vi "S4GUI.vi"(7 "Tab ObsEng":enum32{"Obs", "CCD modes", "Guider", "Eng"}(tab)) -> ()   [LabVIEW 2018] (continued)
        n3771 = call-dynamic "Write # Images.vi"("error in (no error)"=w8549, "# Images"="Exp ch3", "Interface in"=w8552) -> ("error out"=w8497:errorcluster, "Interface out"=w8500:refnum<class "Interface.lvclass">)  [unwired: 7 in]
        n3772 = call-dynamic "ValidateExp.vi"("error in (no error)"=w8497, "Interface in"=w8500) -> ("error out"=w8496:errorcluster, "Interface out"=w8499:refnum<class "Interface.lvclass">)  [unwired: 8 in]
        n3773 = call-dynamic "Read # Images.vi"("error in (no error)"=w8496, "Interface in"=w8499) -> ("error out"=w8495:errorcluster, "# Images"=w8494:u32, "Interface out"=w8498:refnum<class "Interface.lvclass">)  [unwired: 7 in]
        n3774 = call-dynamic "Write #PREV Images.vi"("error in (no error)"=w8495, "#PREV FRAMES"=w8494, "Interface in"=w8498) -> ("error out"=w8548:errorcluster, "Interface out"=w8547:refnum<class "Interface.lvclass">)  [unwired: 7 in]
        n3775 = call-dynamic "Write Interface.vi"("error in (no error)"=w8548, "Interface.lvclass"=w8547, "Channel in"=w8554) -> ("error out"=w8546:errorcluster, "Channel out"=w8553:refnum<class "Channel.lvclass">)  [unwired: 7 in]
        n3776 = property on="Exposures Done ch3" class="Slide (strict)"("Scale.Maximum"=w8494, "Scale.Minimum"=0.0 ("Scale.Range:Minimum")) -> ()  [unwired: 2 in, 2 out]
        n3777 = local write "Exp ch3"(w8494) -> ()
        n3778 = call-dynamic "Write Channel.vi"("error in (no error)"=w8546, "Channel.lvclass"=w8553, "Acquisition in"=w8556) -> ("error out"=w8545:errorcluster, "Acquisition out"=w8555:refnum<class "Acquisition.lvclass">)  [unwired: 7 in]
        n3779 = call-dynamic "Write AcquisitionC.vi"("error in (no error)"=w8545, "Acquisition.lvclass"=w8555, "S4ACS_GUI in"=w8559) -> ("error out"=w8528:errorcluster, "S4ACS_GUI out"=w8529:refnum<class "S4GUI.lvclass">)  [unwired: 7 in]
        n3780 = call-dynamic "Read AcquisitionD.vi"("error in (no error)"=w8528, "S4ACS_GUI in"=w8529) -> ("error out"=w8535:errorcluster, "Acquisition.lvclass"=w8543:refnum<class "Acquisition.lvclass">, "S4ACS_GUI out"=w8544:refnum<class "S4GUI.lvclass">)  [unwired: 7 in]
        n3781 = call-dynamic "Read Channel.vi"("error in (no error)"=w8535, "Acquisition in"=w8543) -> ("error out"=w8536:errorcluster, "Channel.lvclass"=w8542:refnum<class "Channel.lvclass">, "Acquisition out"=w8541:refnum<class "Acquisition.lvclass">)  [unwired: 7 in]
        n3782 = call-dynamic "Read Interface.vi"("error in (no error)"=w8536, "Channel in"=w8542) -> ("error out"=w8534:errorcluster, "Interface.lvclass"=w8537:refnum<class "Interface.lvclass">, "Channel out"=w8539:refnum<class "Channel.lvclass">)  [unwired: 7 in]
        n3783 = call-dynamic "Write # Images.vi"("error in (no error)"=w8534, "# Images"="Exp ch4", "Interface in"=w8537) -> ("error out"=w8488:errorcluster, "Interface out"=w8490:refnum<class "Interface.lvclass">)  [unwired: 7 in]
        n3784 = call-dynamic "ValidateExp.vi"("error in (no error)"=w8488, "Interface in"=w8490) -> ("error out"=w8487:errorcluster, "Interface out"=w8489:refnum<class "Interface.lvclass">)  [unwired: 8 in]
        n3785 = call-dynamic "Read # Images.vi"("error in (no error)"=w8487, "Interface in"=w8489) -> ("error out"=w8492:errorcluster, "# Images"=w8491:u32, "Interface out"=w8493:refnum<class "Interface.lvclass">)  [unwired: 7 in]
        n3786 = call-dynamic "Write #PREV Images.vi"("error in (no error)"=w8492, "#PREV FRAMES"=w8491, "Interface in"=w8493) -> ("error out"=w8533:errorcluster, "Interface out"=w8532:refnum<class "Interface.lvclass">)  [unwired: 7 in]
        n3787 = property on="Exposures Done ch4" class="Slide (strict)"("Scale.Maximum"=w8491, "Scale.Minimum"=0.0 ("Scale.Range:Minimum")) -> ()  [unwired: 2 in, 2 out]
        n3788 = local write "Exp ch4"(w8491) -> ()
        n3789 = call-dynamic "Write Interface.vi"("error in (no error)"=w8533, "Interface.lvclass"=w8532, "Channel in"=w8539) -> ("error out"=w8531:errorcluster, "Channel out"=w8538:refnum<class "Channel.lvclass">)  [unwired: 7 in]
        n3790 = call-dynamic "Write Channel.vi"("error in (no error)"=w8531, "Channel.lvclass"=w8538, "Acquisition in"=w8541) -> ("error out"=w8530:errorcluster, "Acquisition out"=w8540:refnum<class "Acquisition.lvclass">)  [unwired: 7 in]
        n3791 = call-dynamic "Write AcquisitionD.vi"("error in (no error)"=w8530, "Acquisition.lvclass"=w8540, "S4ACS_GUI in"=w8544) -> ("error out"=w8522:errorcluster, "S4ACS_GUI out"=w8523:refnum<class "S4GUI.lvclass">)  [unwired: 7 in]
      }
      event "#cycles ch1": Value Change {
        n3792 = event-data() -> ("NewVal"=w8593:u32)  [unwired: 1 in]
        n3793 = call-dynamic "Read AcquisitionA.vi"("error in (no error)"=w8615, "S4ACS_GUI in"=w8616) -> ("error out"=w8610:errorcluster, "Acquisition.lvclass"=w8613:refnum<class "Acquisition.lvclass">, "S4ACS_GUI out"=w8614:refnum<class "S4GUI.lvclass">)  [unwired: 7 in]
        n3794 = call-dynamic "Read Channel.vi"("error in (no error)"=w8610, "Acquisition in"=w8613) -> ("error out"=w8607:errorcluster, "Channel.lvclass"=w8606:refnum<class "Channel.lvclass">, "Acquisition out"=w8612:refnum<class "Acquisition.lvclass">)  [unwired: 7 in]
        n3795 = call-dynamic "Write ciclos.vi"("error in (no error)"=w8607, "ciclos"=w8593, "Channel in"=w8606) -> ("error out"=w8604:errorcluster, "Channel out"=w8605:refnum<class "Channel.lvclass">)  [unwired: 7 in]
        n3796 = call-dynamic "Write prev ciclos.vi"("error in (no error)"=w8604, "prev ciclos"=w8593, "Channel in"=w8605) -> ("error out"=w8602:errorcluster, "Channel out"=w8603:refnum<class "Channel.lvclass">)  [unwired: 7 in]
        n3797 = property on="Cycles Done ch1" class="Slide (strict)"("Scale.Maximum"=w8593, "Scale.Minimum"=0.0 ("Scale.Range:Minimum")) -> ()  [unwired: 2 in, 2 out]
        n3798 = call-dynamic "Write Channel.vi"("error in (no error)"=w8602, "Channel.lvclass"=w8603, "Acquisition in"=w8612) -> ("error out"=w8609:errorcluster, "Acquisition out"=w8611:refnum<class "Acquisition.lvclass">)  [unwired: 7 in]
        n3799 = call-dynamic "Write AcquisitionA.vi"("error in (no error)"=w8609, "Acquisition.lvclass"=w8611, "S4ACS_GUI in"=w8614) -> ("error out"=w8600:errorcluster, "S4ACS_GUI out"=w8601:refnum<class "S4GUI.lvclass">)  [unwired: 7 in]
        n3800 = call-dynamic "Write ciclos.vi"("error in (no error)"=w8600, "ciclos"=w8593, "S4ACS_GUI in"=w8601) -> ("error out"=w8595:errorcluster, "S4ACS_GUI out"=w8597:refnum<class "S4GUI.lvclass">)  [unwired: 7 in]
        n3801 = call-dynamic "Write prev sequencias.vi"("error in (no error)"=w8595, "prev sequencias"=w8593, "S4GUI in"=w8597) -> ("error out"=w8594:errorcluster, "S4GUI out"=w8596:refnum<class "S4GUI.lvclass">)  [unwired: 7 in]
        n3802 = call-dynamic "Write TotalCiclos.vi"("error in (no error)"=w8594, "TotalCiclos"=w8593, "S4GUI in"=w8596) -> ("error out"=w8598:errorcluster, "S4GUI out"=w8599:refnum<class "S4GUI.lvclass">)  [unwired: 7 in]
      }
      event "#cycles ch2": Value Change {
        n3803 = event-data() -> ("NewVal"=w8617:u32)  [unwired: 1 in]
        n3804 = call "Read AcquisitionB.vi"("error in (no error)"=w8639, "S4ACS_GUI in"=w8640) -> ("error out"=w8634:errorcluster, "Acquisition.lvclass"=w8637:refnum<class "Acquisition.lvclass">, "S4ACS_GUI out"=w8638:refnum<class "S4GUI.lvclass">)  [unwired: 7 in]
        n3805 = call-dynamic "Read Channel.vi"("error in (no error)"=w8634, "Acquisition in"=w8637) -> ("error out"=w8632:errorcluster, "Channel.lvclass"=w8631:refnum<class "Channel.lvclass">, "Acquisition out"=w8636:refnum<class "Acquisition.lvclass">)  [unwired: 7 in]
        n3806 = call-dynamic "Write ciclos.vi"("error in (no error)"=w8632, "ciclos"=w8617, "Channel in"=w8631) -> ("error out"=w8629:errorcluster, "Channel out"=w8630:refnum<class "Channel.lvclass">)  [unwired: 7 in]
        n3807 = call-dynamic "Write prev ciclos.vi"("error in (no error)"=w8629, "prev ciclos"=w8617, "Channel in"=w8630) -> ("error out"=w8627:errorcluster, "Channel out"=w8628:refnum<class "Channel.lvclass">)  [unwired: 7 in]
        n3808 = call-dynamic "Write Channel.vi"("error in (no error)"=w8627, "Channel.lvclass"=w8628, "Acquisition in"=w8636) -> ("error out"=w8633:errorcluster, "Acquisition out"=w8635:refnum<class "Acquisition.lvclass">)  [unwired: 7 in]
        n3809 = property on="Cycles Done ch2" class="Slide (strict)"("Scale.Maximum"=w8617, "Scale.Minimum"=0.0 ("Scale.Range:Minimum")) -> ()  [unwired: 2 in, 2 out]
        n3810 = call "Write AcquisitionB.vi"("error in (no error)"=w8633, "Acquisition.lvclass"=w8635, "S4ACS_GUI in"=w8638) -> ("error out"=w8625:errorcluster, "S4ACS_GUI out"=w8626:refnum<class "S4GUI.lvclass">)  [unwired: 7 in]
        n3811 = call-dynamic "Write ciclos.vi"("error in (no error)"=w8625, "ciclos"=w8617, "S4ACS_GUI in"=w8626) -> ("error out"=w8620:errorcluster, "S4ACS_GUI out"=w8622:refnum<class "S4GUI.lvclass">)  [unwired: 7 in]
        n3812 = call-dynamic "Write prev sequencias.vi"("error in (no error)"=w8620, "prev sequencias"=w8617, "S4GUI in"=w8622) -> ("error out"=w8619:errorcluster, "S4GUI out"=w8621:refnum<class "S4GUI.lvclass">)  [unwired: 7 in]
        n3813 = call-dynamic "Write TotalCiclos.vi"("error in (no error)"=w8619, "TotalCiclos"=w8617, "S4GUI in"=w8621) -> ("error out"=w8623:errorcluster, "S4GUI out"=w8624:refnum<class "S4GUI.lvclass">)  [unwired: 7 in]
      }
      event "#cycles ch3": Value Change {
        n3814 = event-data() -> ("NewVal"=w8641:u32)  [unwired: 1 in]
        n3815 = call-dynamic "Read AcquisitionC.vi"("error in (no error)"=w8663, "S4ACS_GUI in"=w8664) -> ("error out"=w8658:errorcluster, "Acquisition.lvclass"=w8661:refnum<class "Acquisition.lvclass">, "S4ACS_GUI out"=w8662:refnum<class "S4GUI.lvclass">)  [unwired: 7 in]
        n3816 = call-dynamic "Read Channel.vi"("error in (no error)"=w8658, "Acquisition in"=w8661) -> ("error out"=w8656:errorcluster, "Channel.lvclass"=w8655:refnum<class "Channel.lvclass">, "Acquisition out"=w8660:refnum<class "Acquisition.lvclass">)  [unwired: 7 in]
        n3817 = call-dynamic "Write ciclos.vi"("error in (no error)"=w8656, "ciclos"=w8641, "Channel in"=w8655) -> ("error out"=w8653:errorcluster, "Channel out"=w8654:refnum<class "Channel.lvclass">)  [unwired: 7 in]
        n3818 = call-dynamic "Write prev ciclos.vi"("error in (no error)"=w8653, "prev ciclos"=w8641, "Channel in"=w8654) -> ("error out"=w8651:errorcluster, "Channel out"=w8652:refnum<class "Channel.lvclass">)  [unwired: 7 in]
        n3819 = call-dynamic "Write Channel.vi"("error in (no error)"=w8651, "Channel.lvclass"=w8652, "Acquisition in"=w8660) -> ("error out"=w8657:errorcluster, "Acquisition out"=w8659:refnum<class "Acquisition.lvclass">)  [unwired: 7 in]
        n3820 = property on="Cycles Done ch3" class="Slide (strict)"("Scale.Maximum"=w8641, "Scale.Minimum"=0.0 ("Scale.Range:Minimum")) -> ()  [unwired: 2 in, 2 out]
        n3821 = call-dynamic "Write AcquisitionC.vi"("error in (no error)"=w8657, "Acquisition.lvclass"=w8659, "S4ACS_GUI in"=w8662) -> ("error out"=w8649:errorcluster, "S4ACS_GUI out"=w8650:refnum<class "S4GUI.lvclass">)  [unwired: 7 in]
        n3822 = call-dynamic "Write ciclos.vi"("error in (no error)"=w8649, "ciclos"=w8641, "S4ACS_GUI in"=w8650) -> ("error out"=w8644:errorcluster, "S4ACS_GUI out"=w8646:refnum<class "S4GUI.lvclass">)  [unwired: 7 in]
        n3823 = call-dynamic "Write prev sequencias.vi"("error in (no error)"=w8644, "prev sequencias"=w8641, "S4GUI in"=w8646) -> ("error out"=w8643:errorcluster, "S4GUI out"=w8645:refnum<class "S4GUI.lvclass">)  [unwired: 7 in]
        n3824 = call-dynamic "Write TotalCiclos.vi"("error in (no error)"=w8643, "TotalCiclos"=w8641, "S4GUI in"=w8645) -> ("error out"=w8647:errorcluster, "S4GUI out"=w8648:refnum<class "S4GUI.lvclass">)  [unwired: 7 in]
      }
      event "#cycles ch4": Value Change {
        n3825 = event-data() -> ("NewVal"=w8665:u32)  [unwired: 1 in]
        n3826 = call-dynamic "Read AcquisitionD.vi"("error in (no error)"=w8687, "S4ACS_GUI in"=w8688) -> ("error out"=w8682:errorcluster, "Acquisition.lvclass"=w8685:refnum<class "Acquisition.lvclass">, "S4ACS_GUI out"=w8686:refnum<class "S4GUI.lvclass">)  [unwired: 7 in]
        n3827 = call-dynamic "Read Channel.vi"("error in (no error)"=w8682, "Acquisition in"=w8685) -> ("error out"=w8680:errorcluster, "Channel.lvclass"=w8679:refnum<class "Channel.lvclass">, "Acquisition out"=w8684:refnum<class "Acquisition.lvclass">)  [unwired: 7 in]
        n3828 = call-dynamic "Write ciclos.vi"("error in (no error)"=w8680, "ciclos"=w8665, "Channel in"=w8679) -> ("error out"=w8677:errorcluster, "Channel out"=w8678:refnum<class "Channel.lvclass">)  [unwired: 7 in]
        n3829 = call-dynamic "Write prev ciclos.vi"("error in (no error)"=w8677, "prev ciclos"=w8665, "Channel in"=w8678) -> ("error out"=w8675:errorcluster, "Channel out"=w8676:refnum<class "Channel.lvclass">)  [unwired: 7 in]
        n3830 = call-dynamic "Write Channel.vi"("error in (no error)"=w8675, "Channel.lvclass"=w8676, "Acquisition in"=w8684) -> ("error out"=w8681:errorcluster, "Acquisition out"=w8683:refnum<class "Acquisition.lvclass">)  [unwired: 7 in]
        n3831 = call-dynamic "Write AcquisitionD.vi"("error in (no error)"=w8681, "Acquisition.lvclass"=w8683, "S4ACS_GUI in"=w8686) -> ("error out"=w8673:errorcluster, "S4ACS_GUI out"=w8674:refnum<class "S4GUI.lvclass">)  [unwired: 7 in]
        n3832 = property on="Cycles Done ch4" class="Slide (strict)"("Scale.Maximum"=w8665, "Scale.Minimum"=0.0 ("Scale.Range:Minimum")) -> ()  [unwired: 2 in, 2 out]
        n3833 = call-dynamic "Write ciclos.vi"("error in (no error)"=w8673, "ciclos"=w8665, "S4ACS_GUI in"=w8674) -> ("error out"=w8668:errorcluster, "S4ACS_GUI out"=w8670:refnum<class "S4GUI.lvclass">)  [unwired: 7 in]
        n3834 = call-dynamic "Write prev sequencias.vi"("error in (no error)"=w8668, "prev sequencias"=w8665, "S4GUI in"=w8670) -> ("error out"=w8667:errorcluster, "S4GUI out"=w8669:refnum<class "S4GUI.lvclass">)  [unwired: 7 in]
        n3835 = call-dynamic "Write TotalCiclos.vi"("error in (no error)"=w8667, "TotalCiclos"=w8665, "S4GUI in"=w8669) -> ("error out"=w8671:errorcluster, "S4GUI out"=w8672:refnum<class "S4GUI.lvclass">)  [unwired: 7 in]
      }
      event "Start ch2": Value Change {
        n3836 = event-data() -> ()  [unwired: 1 in, 6 out]
        n3837 = call "Read Instrument.lvclass.vi"("error in (no error)"=w8702, "S4ACS_GUI in"=w8703) -> ("error out"=w8704:errorcluster, "Instrument.lvclass"=w8705:refnum<class "Instrument.lvclass">, "S4ACS_GUI out"=w8701:refnum<class "S4GUI.lvclass">)  [unwired: 7 in]
        n3838 = call-dynamic "Read mode.vi"("error in (no error)"=w8704, "Instrument in"=w8705) -> ("error out"=w8700:errorcluster, "mode"=w8699:bool)  [unwired: 7 in, 1 out]
        n3839 = call "Read AcquisitionB.vi"("error in (no error)"=w8700, "S4ACS_GUI in"=w8701) -> ("error out"=w8717:errorcluster, "Acquisition.lvclass"=w8718:refnum<class "Acquisition.lvclass">, "S4ACS_GUI out"=w8720:refnum<class "S4GUI.lvclass">)  [unwired: 7 in]
        n3840 = call-dynamic "Read Acq_state.vi"("error in (no error)"=w8717, "Acquisition in"=w8718) -> ("error out"=w8714:errorcluster, "Acq_state"=w8716:u32, "Acquisition out"=w8713:refnum<class "Acquisition.lvclass">)  [unwired: 7 in]
        n3841 = Not Equal?(x=w8716, y=u32 400) -> (x != y?=w8719:bool)
        n3842 = case shown="True" w8719 {
          tunnel: w8720 -> [w8733 w8772]
          tunnel: [w8733 w8764] -> w8712
          tunnel: [w8728 w8754] -> w8698
          tunnel: w8714 -> [w8735 w8762]
          tunnel: w8713 -> [w8738 w8765]
          tunnel: [w8729 w8753] -> w8711
          tunnel: w8710 -> [_ w8786]
          tunnel: w8709 -> [_ w8785]
          tunnel: w8708 -> [_ w8784]
          tunnel: w8707 -> [_ w8783]
          tunnel: w8706 -> [_ w8777]
          tunnel: w8699 -> [_ _]
          tunnel: w8697 -> [_ w8760]
          tunnel: w8696 -> [_ w8759]
          tunnel: w8695 -> [_ w8758]
          tunnel: w8694 -> [_ w8757]
          frame False {
            n3843 = call-dynamic "Read Acq_prevstate.vi"("error in (no error)"=w8735, "Acquisition in"=w8738) -> ("error out"=w8734:errorcluster, "Acq_prevstate"=w8736:u32, "Acquisition out"=w8737:refnum<class "Acquisition.lvclass">)  [unwired: 7 in]
            n3844 = call-dynamic "Write Acq_state.vi"("error in (no error)"=w8734, "Acq_state"=w8736, "Acquisition in"=w8737) -> ("error out"=w8725:errorcluster, "Acquisition out"=w8727:refnum<class "Acquisition.lvclass">)  [unwired: 7 in]
            n3845 = call-dynamic "Read enabled.vi"("error in (no error)"=w8725, "Server in"=w8727) -> ("error out"=w8724:errorcluster, "enabled"=w8721:bool, "Server out"=w8726:refnum<class "Acquisition.lvclass">)  [unwired: 7 in]
            n3846 = call-dynamic "Read Channel.vi"("error in (no error)"=w8724, "Acquisition in"=w8726) -> ("error out"=w8722:errorcluster, "Channel.lvclass"=w8723:refnum<class "Channel.lvclass">, "Acquisition out"=w8732:refnum<class "Acquisition.lvclass">)  [unwired: 7 in]
            n3847 = case shown="True" w8721 {
              tunnel: w8723 -> [w8740 w8750]
              tunnel: [w8740 w8748] -> w8731
              tunnel: w8722 -> [w8739 w8745]
              tunnel: [w8739 w8743] -> w8730
              frame False {
              }
              frame True {
                n3848 = call-dynamic "Read State Machine.vi"("error in (no error)"=w8745, "Device in"=w8750) -> ("error out"=w8741:errorcluster, "State Machine.lvclass"=w8742:refnum<class "State Machine.lvclass">, "Device out"=w8749:refnum<class "Channel.lvclass">)  [unwired: 7 in]
                n3849 = call "Next State.vi"("error in (no error)"=w8741, "New_State"=96, "State Machine in"=w8742) -> ("error out"=w8744:errorcluster, "State Machine out"=w8747:refnum<class "State Machine.lvclass">)  [unwired: 7 in]
                n3850 = call-dynamic "Write State Machine.vi"("error in (no error)"=w8744, "State Machine.lvclass"=w8747, "Device in"=w8749) -> ("error out"=w8743:errorcluster, "Device out"=w8748:refnum<class "Channel.lvclass">)  [unwired: 7 in]
              }
            }
            n3851 = call-dynamic "Write Channel.vi"("error in (no error)"=w8730, "Channel.lvclass"=w8731, "Acquisition in"=w8732) -> ("error out"=w8728:errorcluster, "Acquisition out"=w8729:refnum<class "Acquisition.lvclass">)  [unwired: 7 in]
          }
          frame True {
            # "obs type"
            # "suffix"
            # "object"
            n3852 = call "Read Instrument.lvclass.vi"("S4ACS_GUI in"=w8772) -> ("error out"=w8774:errorcluster, "Instrument.lvclass"=w8776:refnum<class "Instrument.lvclass">, "S4ACS_GUI out"=w8766:refnum<class "S4GUI.lvclass">)  [unwired: 8 in]
            n3853 = call "Read WPROT.vi"("error in (no error)"=w8774, "Instrument in"=w8776) -> ("error out"=w8773:errorcluster, "Opt_Selector.lvclass"=w8775:refnum<class "Opt_Selector.lvclass">)  [unwired: 7 in, 1 out]
            n3854 = call-dynamic "Read sequencia.vi"("error in (no error)"=w8773, "Opt_Selector in"=w8775) -> ()  [unwired: 7 in, 3 out]
            n3855 = case shown="Default" w8760 {
              tunnel: [u32 271 ("Obs_state") u32 251 ("Obs_state")] -> w8763
              tunnel: w8762 -> [w8811 w8822]
              tunnel: [w8810 w8822] -> w8761
              tunnel: w8759 -> [w8818 _]
              tunnel: w8758 -> [w8817 _]
              tunnel: w8757 -> [w8816 _]
              tunnel: w8766 -> [w8809 w8821]
              tunnel: [w8808 w8821] -> w8764
              frame "FOCUS" {
                n3856 = call-dynamic "Read TelFocus.lvclass.vi"("error in (no error)"=w8811, "S4GUI in"=w8809) -> ("error out"=w8813:errorcluster, "TelFocus.lvclass"=w8815:refnum<class "TelFocus.lvclass">, "S4GUI out"=w8819:refnum<class "S4GUI.lvclass">)  [unwired: 7 in]
                n3857 = call-dynamic "LoadParam.vi"("#steps"=w8816, "error in (no error)"=w8813, "step"=w8817, "init"=w8818, "TelFocus in"=w8815) -> ("error out"=w8812:errorcluster, "TelFocus out"=w8814:refnum<class "TelFocus.lvclass">)  [unwired: 5 in]
                n3858 = call-dynamic "Write TelFocus.lvclass.vi"("error in (no error)"=w8812, "TelFocus.lvclass"=w8814, "S4GUI in"=w8819) -> ("error out"=w8810:errorcluster, "S4GUI out"=w8808:refnum<class "S4GUI.lvclass">)  [unwired: 7 in]
              }
              frame Default {
              }
            }
            n3859 = property on="Start ch2" class="Bool"(error in=w8762, "DisabledEnum"=T12."Disabled and Grayed Out" ("Disabled")) -> ()  [unwired: 1 in, 2 out]
            n3860 = call-dynamic "Write Acq_state.vi"("error in (no error)"=w8761, "Acq_state"=w8763, "Acquisition in"=w8765) -> ("error out"=w8787:errorcluster, "Acquisition out"=w8788:refnum<class "Acquisition.lvclass">)  [unwired: 7 in]
            n3861 = call-dynamic "Read Channel.vi"("error in (no error)"=w8787, "Acquisition in"=w8788) -> ("error out"=w8789:errorcluster, "Channel.lvclass"=w8790:refnum<class "Channel.lvclass">, "Acquisition out"=w8794:refnum<class "Acquisition.lvclass">)  [unwired: 7 in]
            n3862 = call-dynamic "Read Interface.vi"("error in (no error)"=w8789, "Channel in"=w8790) -> ("error out"=w8806:errorcluster, "Interface.lvclass"=w8807:refnum<class "Interface.lvclass">, "Channel out"=w8805:refnum<class "Channel.lvclass">)  [unwired: 7 in]
            n3863 = call "Write Exposure Time.vi"("error in (no error)"=w8806, "Exposure Time"="Exptime ch2", "Interface in"=w8807) -> ("error out"=w8769:errorcluster, "Interface out"=w8771:refnum<class "Interface.lvclass">)  [unwired: 7 in]
            n3864 = case shown="Default" w8760 {
              tunnel: w8771 -> [w8825 w8830]
              tunnel: [w8825 w8829] -> w8770
              tunnel: w8769 -> [w8824 w8828]
              tunnel: [w8824 w8827] -> w8768
              tunnel: "Exptime ch2" -> [_ w8826]
              frame "ZERO" {
              }
              frame Default {
                n3865 = call-dynamic "Write prev ExpTime.vi"("error in (no error)"=w8828, "prev ExpTime"=w8826, "Interface in"=w8830) -> ("error out"=w8827:errorcluster, "Interface out"=w8829:refnum<class "Interface.lvclass">)  [unwired: 7 in]
              }
            }
            n3866 = call-dynamic "Write # Index.vi"("error in (no error)"=w8768, "# Index"="Index ch2", "Interface in"=w8770) -> ("error out"=w8803:errorcluster, "Interface out"=w8804:refnum<class "Interface.lvclass">)  [unwired: 7 in]
            n3867 = call-dynamic "Write Suffix.vi"("error in (no error)"=w8803, "Suffix"=w8786, "Interface in"=w8804) -> ("error out"=w8802:errorcluster, "Interface out"=w8801:refnum<class "Interface.lvclass">)  [unwired: 7 in]
            n3868 = call-dynamic "Write ObsType.vi"("error in (no error)"=w8802, "ObsType"=w8784, "Interface in"=w8801) -> ("error out"=w8799:errorcluster, "Interface out"=w8800:refnum<class "Interface.lvclass">)  [unwired: 7 in]
            n3869 = call-dynamic "Write Object.vi"("error in (no error)"=w8799, "Object"=w8783, "Interface in"=w8800) -> ("error out"=w8798:errorcluster, "Interface out"=w8797:refnum<class "Interface.lvclass">)  [unwired: 7 in]
            n3870 = call-dynamic "Write Comments.vi"("error in (no error)"=w8798, "Comments"=w8785, "Interface in"=w8797) -> ("error out"=w8795:errorcluster, "Interface out"=w8796:refnum<class "Interface.lvclass">)  [unwired: 7 in]
            n3871 = call-dynamic "Write DS9.vi"("error in (no error)"=w8795, "DS9"="F", "Interface in"=w8796) -> ("error out"=w8780:errorcluster, "Interface out"=w8782:refnum<class "Interface.lvclass">)  [unwired: 7 in]
            n3872 = call-dynamic "Write Observer.vi"("error in (no error)"=w8780, "Observer"=w8777, "Interface in"=w8782) -> ("error out"=w8779:errorcluster, "Interface out"=w8781:refnum<class "Interface.lvclass">)  [unwired: 7 in]
            n3873 = property on="Exposure Time ch2" class="Slide (strict)"("Scale.Maximum"="Exptime ch2", "Scale.Minimum"=0.0 ("Scale.Range:Minimum")) -> ()  [unwired: 2 in, 2 out]
            n3874 = call-dynamic "Write Interface.vi"("error in (no error)"=w8779, "Interface.lvclass"=w8781, "Channel in"=w8805) -> ("error out"=w8751:errorcluster, "Channel out"=w8752:refnum<class "Channel.lvclass">)  [unwired: 7 in]
            n3875 = call-dynamic "Write Channel.vi"("error in (no error)"=w8751, "Channel.lvclass"=w8752, "Acquisition in"=w8794) -> ("error out"=w8755:errorcluster, "Acquisition out"=w8756:refnum<class "Acquisition.lvclass">)  [unwired: 7 in]
            n3876 = call-dynamic "CalcCubeDuration.vi"("error in (no error)"=w8755, "Acquisition in"=w8756) -> ("error out"=w8754:errorcluster, "Acquisition out"=w8753:refnum<class "Acquisition.lvclass">)  [unwired: 8 in]
          }
        }
        n3877 = call "Write AcquisitionB.vi"("error in (no error)"=w8698, "Acquisition.lvclass"=w8711, "S4ACS_GUI in"=w8712) -> ("error out"=w8691:errorcluster, "S4ACS_GUI out"=w8692:refnum<class "S4GUI.lvclass">)  [unwired: 7 in]
        n3878 = call-dynamic "Write User Event.vi"("error in (no error)"=w8691, "User Event"="START ASYNC CH2", "S4GUI in"=w8692) -> ("error out"=w8689:errorcluster, "S4GUI out"=w8690:refnum<class "S4GUI.lvclass">)  [unwired: 7 in]
      }
      event "Start ch3": Value Change {
        n3879 = event-data() -> ()  [unwired: 1 in, 6 out]
        n3880 = call "Read Instrument.lvclass.vi"("error in (no error)"=w8843, "S4ACS_GUI in"=w8845) -> ("error out"=w8846:errorcluster, "Instrument.lvclass"=w8847:refnum<class "Instrument.lvclass">, "S4ACS_GUI out"=w8844:refnum<class "S4GUI.lvclass">)  [unwired: 7 in]
        n3881 = call-dynamic "Read mode.vi"("error in (no error)"=w8846, "Instrument in"=w8847) -> ("error out"=w8842:errorcluster, "mode"=w8841:bool)  [unwired: 7 in, 1 out]
        n3882 = call-dynamic "Read AcquisitionC.vi"("error in (no error)"=w8842, "S4ACS_GUI in"=w8844) -> ("error out"=w8859:errorcluster, "Acquisition.lvclass"=w8860:refnum<class "Acquisition.lvclass">, "S4ACS_GUI out"=w8862:refnum<class "S4GUI.lvclass">)  [unwired: 7 in]
        n3883 = call-dynamic "Read Acq_state.vi"("error in (no error)"=w8859, "Acquisition in"=w8860) -> ("error out"=w8856:errorcluster, "Acq_state"=w8858:u32, "Acquisition out"=w8855:refnum<class "Acquisition.lvclass">)  [unwired: 7 in]
        n3884 = Not Equal?(x=w8858, y=u32 400) -> (x != y?=w8861:bool)
        n3885 = case shown="True" w8861 {
          tunnel: w8862 -> [w8875 w8911]
          tunnel: [w8875 w8902] -> w8854
          tunnel: [w8870 w8894] -> w8840
          tunnel: w8856 -> [w8877 w8904]
          tunnel: w8855 -> [w8880 w8905]
          tunnel: [w8871 w8893] -> w8853
          tunnel: w8852 -> [_ w8924]
          tunnel: w8851 -> [_ w8923]
          tunnel: w8850 -> [_ w8922]
          tunnel: w8849 -> [_ w8921]
          tunnel: w8848 -> [_ w8916]
          tunnel: w8841 -> [_ _]
          tunnel: w8839 -> [_ w8900]
          tunnel: w8838 -> [_ w8899]
          tunnel: w8837 -> [_ w8898]
          tunnel: w8836 -> [_ w8897]
          frame False {
            n3886 = call-dynamic "Read Acq_prevstate.vi"("error in (no error)"=w8877, "Acquisition in"=w8880) -> ("error out"=w8876:errorcluster, "Acq_prevstate"=w8878:u32, "Acquisition out"=w8879:refnum<class "Acquisition.lvclass">)  [unwired: 7 in]
            n3887 = call-dynamic "Write Acq_state.vi"("error in (no error)"=w8876, "Acq_state"=w8878, "Acquisition in"=w8879) -> ("error out"=w8865:errorcluster, "Acquisition out"=w8867:refnum<class "Acquisition.lvclass">)  [unwired: 7 in]
            n3888 = call-dynamic "Read enabled.vi"("error in (no error)"=w8865, "Server in"=w8867) -> ("error out"=w8864:errorcluster, "enabled"=w8863:bool, "Server out"=w8866:refnum<class "Acquisition.lvclass">)  [unwired: 7 in]
            n3889 = call-dynamic "Read Channel.vi"("error in (no error)"=w8864, "Acquisition in"=w8866) -> ("error out"=w8868:errorcluster, "Channel.lvclass"=w8869:refnum<class "Channel.lvclass">, "Acquisition out"=w8873:refnum<class "Acquisition.lvclass">)  [unwired: 7 in]
            n3890 = case shown="True" w8863 {
              tunnel: w8869 -> [w8882 w8892]
              tunnel: [w8882 w8890] -> w8872
              tunnel: w8868 -> [w8881 w8887]
              tunnel: [w8881 w8885] -> w8874
              frame False {
              }
              frame True {
                n3891 = call-dynamic "Read State Machine.vi"("error in (no error)"=w8887, "Device in"=w8892) -> ("error out"=w8883:errorcluster, "State Machine.lvclass"=w8884:refnum<class "State Machine.lvclass">, "Device out"=w8891:refnum<class "Channel.lvclass">)  [unwired: 7 in]
                n3892 = call "Next State.vi"("error in (no error)"=w8883, "New_State"=96, "State Machine in"=w8884) -> ("error out"=w8886:errorcluster, "State Machine out"=w8889:refnum<class "State Machine.lvclass">)  [unwired: 7 in]
                n3893 = call-dynamic "Write State Machine.vi"("error in (no error)"=w8886, "State Machine.lvclass"=w8889, "Device in"=w8891) -> ("error out"=w8885:errorcluster, "Device out"=w8890:refnum<class "Channel.lvclass">)  [unwired: 7 in]
              }
            }
            n3894 = call-dynamic "Write Channel.vi"("error in (no error)"=w8874, "Channel.lvclass"=w8872, "Acquisition in"=w8873) -> ("error out"=w8870:errorcluster, "Acquisition out"=w8871:refnum<class "Acquisition.lvclass">)  [unwired: 7 in]
          }
          frame True {
            # "obs type"
            # "suffix"
            # "object"
            n3895 = call "Read Instrument.lvclass.vi"("S4ACS_GUI in"=w8911) -> ("error out"=w8913:errorcluster, "Instrument.lvclass"=w8915:refnum<class "Instrument.lvclass">, "S4ACS_GUI out"=w8903:refnum<class "S4GUI.lvclass">)  [unwired: 8 in]
            n3896 = call "Read WPROT.vi"("error in (no error)"=w8913, "Instrument in"=w8915) -> ("error out"=w8912:errorcluster, "Opt_Selector.lvclass"=w8914:refnum<class "Opt_Selector.lvclass">)  [unwired: 7 in, 1 out]
            n3897 = call-dynamic "Read sequencia.vi"("error in (no error)"=w8912, "Opt_Selector in"=w8914) -> ()  [unwired: 7 in, 3 out]
            n3898 = case shown="\"FOCUS\"" w8900 {
              tunnel: [u32 271 ("Obs_state") u32 251 ("Obs_state")] -> w8901
              tunnel: w8904 -> [w8952 w8963]
              tunnel: [w8951 w8963] -> _
              tunnel: w8899 -> [w8959 _]
              tunnel: w8898 -> [w8958 _]
              tunnel: w8897 -> [w8957 _]
              tunnel: w8903 -> [w8950 w8962]
              tunnel: [w8949 w8962] -> w8902
              frame "FOCUS" {
                n3899 = call-dynamic "Read TelFocus.lvclass.vi"("error in (no error)"=w8952, "S4GUI in"=w8950) -> ("error out"=w8954:errorcluster, "TelFocus.lvclass"=w8956:refnum<class "TelFocus.lvclass">, "S4GUI out"=w8960:refnum<class "S4GUI.lvclass">)  [unwired: 7 in]
                n3900 = call-dynamic "LoadParam.vi"("#steps"=w8957, "error in (no error)"=w8954, "step"=w8958, "init"=w8959, "TelFocus in"=w8956) -> ("error out"=w8953:errorcluster, "TelFocus out"=w8955:refnum<class "TelFocus.lvclass">)  [unwired: 5 in]
                n3901 = call-dynamic "Write TelFocus.lvclass.vi"("error in (no error)"=w8953, "TelFocus.lvclass"=w8955, "S4GUI in"=w8960) -> ("error out"=w8951:errorcluster, "S4GUI out"=w8949:refnum<class "S4GUI.lvclass">)  [unwired: 7 in]
              }
              frame Default {
              }
            }
            n3902 = call-dynamic "Write Acq_state.vi"("Acq_state"=w8901, "Acquisition in"=w8905) -> ("error out"=w8925:errorcluster, "Acquisition out"=w8926:refnum<class "Acquisition.lvclass">)  [unwired: 8 in]
            n3903 = call-dynamic "Read Channel.vi"("error in (no error)"=w8925, "Acquisition in"=w8926) -> ("error out"=w8927:errorcluster, "Channel.lvclass"=w8928:refnum<class "Channel.lvclass">, "Acquisition out"=w8935:refnum<class "Acquisition.lvclass">)  [unwired: 7 in]
            n3904 = property on="Start ch3" class="Bool"(error in=w8904, "DisabledEnum"=T12."Disabled and Grayed Out" ("Disabled")) -> ()  [unwired: 1 in, 2 out]
            n3905 = call-dynamic "Read Interface.vi"("error in (no error)"=w8927, "Channel in"=w8928) -> ("error out"=w8947:errorcluster, "Interface.lvclass"=w8948:refnum<class "Interface.lvclass">, "Channel out"=w8946:refnum<class "Channel.lvclass">)  [unwired: 7 in]
            n3906 = call "Write Exposure Time.vi"("error in (no error)"=w8947, "Exposure Time"="Exptime ch3", "Interface in"=w8948) -> ("error out"=w8908:errorcluster, "Interface out"=w8909:refnum<class "Interface.lvclass">)  [unwired: 7 in]
            n3907 = case shown="\"ZERO\"" w8900 {
              tunnel: [w8965 w8971] -> w8910
              tunnel: w8909 -> [w8965 w8970]
              tunnel: w8908 -> [w8966 w8969]
              tunnel: [w8966 w8968] -> w8907
              tunnel: "Exptime ch3" -> [_ w8967]
              frame "ZERO" {
              }
              frame Default {
                n3908 = call-dynamic "Write prev ExpTime.vi"("error in (no error)"=w8969, "prev ExpTime"=w8967, "Interface in"=w8970) -> ("error out"=w8968:errorcluster, "Interface out"=w8971:refnum<class "Interface.lvclass">)  [unwired: 7 in]
              }
            }
            n3909 = call-dynamic "Write # Index.vi"("error in (no error)"=w8907, "# Index"="Index ch3", "Interface in"=w8910) -> ("error out"=w8944:errorcluster, "Interface out"=w8945:refnum<class "Interface.lvclass">)  [unwired: 7 in]
            n3910 = call-dynamic "Write Suffix.vi"("error in (no error)"=w8944, "Suffix"=w8924, "Interface in"=w8945) -> ("error out"=w8943:errorcluster, "Interface out"=w8942:refnum<class "Interface.lvclass">)  [unwired: 7 in]
            n3911 = call-dynamic "Write ObsType.vi"("error in (no error)"=w8943, "ObsType"=w8921, "Interface in"=w8942) -> ("error out"=w8940:errorcluster, "Interface out"=w8941:refnum<class "Interface.lvclass">)  [unwired: 7 in]
            n3912 = call-dynamic "Write Object.vi"("error in (no error)"=w8940, "Object"=w8922, "Interface in"=w8941) -> ("error out"=w8939:errorcluster, "Interface out"=w8938:refnum<class "Interface.lvclass">)  [unwired: 7 in]
            n3913 = call-dynamic "Write Comments.vi"("error in (no error)"=w8939, "Comments"=w8923, "Interface in"=w8938) -> ("error out"=w8936:errorcluster, "Interface out"=w8937:refnum<class "Interface.lvclass">)  [unwired: 7 in]
            n3914 = call-dynamic "Write DS9.vi"("error in (no error)"=w8936, "DS9"="F", "Interface in"=w8937) -> ("error out"=w8918:errorcluster, "Interface out"=w8920:refnum<class "Interface.lvclass">)  [unwired: 7 in]
            n3915 = call-dynamic "Write Observer.vi"("error in (no error)"=w8918, "Observer"=w8916, "Interface in"=w8920) -> ("error out"=w8917:errorcluster, "Interface out"=w8919:refnum<class "Interface.lvclass">)  [unwired: 7 in]
            n3916 = call-dynamic "Write Interface.vi"("error in (no error)"=w8917, "Interface.lvclass"=w8919, "Channel in"=w8946) -> ("error out"=w8929:errorcluster, "Channel out"=w8930:refnum<class "Channel.lvclass">)  [unwired: 7 in]
            n3917 = property on="Exposure Time ch3" class="Slide (strict)"("Scale.Maximum"="Exptime ch3", "Scale.Minimum"=0.0 ("Scale.Range:Minimum")) -> ()  [unwired: 2 in, 2 out]
            n3918 = call-dynamic "Write Channel.vi"("error in (no error)"=w8929, "Channel.lvclass"=w8930, "Acquisition in"=w8935) -> ("error out"=w8895:errorcluster, "Acquisition out"=w8896:refnum<class "Acquisition.lvclass">)  [unwired: 7 in]
            n3919 = call-dynamic "CalcCubeDuration.vi"("error in (no error)"=w8895, "Acquisition in"=w8896) -> ("error out"=w8894:errorcluster, "Acquisition out"=w8893:refnum<class "Acquisition.lvclass">)  [unwired: 8 in]
          }
        }
        n3920 = call-dynamic "Write AcquisitionC.vi"("error in (no error)"=w8840, "Acquisition.lvclass"=w8853, "S4ACS_GUI in"=w8854) -> ("error out"=w8833:errorcluster, "S4ACS_GUI out"=w8834:refnum<class "S4GUI.lvclass">)  [unwired: 7 in]
        n3921 = call-dynamic "Write User Event.vi"("error in (no error)"=w8833, "User Event"="START ASYNC CH3", "S4GUI in"=w8834) -> ("error out"=w8832:errorcluster, "S4GUI out"=w8831:refnum<class "S4GUI.lvclass">)  [unwired: 7 in]
      }
      event "Start ch4": Value Change {
        n3922 = event-data() -> ()  [unwired: 1 in, 6 out]
        n3923 = call "Read Instrument.lvclass.vi"("error in (no error)"=w8986, "S4ACS_GUI in"=w8987) -> ("error out"=w8988:errorcluster, "Instrument.lvclass"=w8989:refnum<class "Instrument.lvclass">, "S4ACS_GUI out"=w8985:refnum<class "S4GUI.lvclass">)  [unwired: 7 in]
        n3924 = call-dynamic "Read mode.vi"("error in (no error)"=w8988, "Instrument in"=w8989) -> ("error out"=w8984:errorcluster, "mode"=w8983:bool)  [unwired: 7 in, 1 out]
        n3925 = call-dynamic "Read AcquisitionD.vi"("error in (no error)"=w8984, "S4ACS_GUI in"=w8985) -> ("error out"=w9000:errorcluster, "Acquisition.lvclass"=w9001:refnum<class "Acquisition.lvclass">, "S4ACS_GUI out"=w9003:refnum<class "S4GUI.lvclass">)  [unwired: 7 in]
        n3926 = call-dynamic "Read Acq_state.vi"("error in (no error)"=w9000, "Acquisition in"=w9001) -> ("error out"=w8997:errorcluster, "Acq_state"=w8999:u32, "Acquisition out"=w8996:refnum<class "Acquisition.lvclass">)  [unwired: 7 in]
        n3927 = Not Equal?(x=w8999, y=u32 400) -> (x != y?=w9002:bool)
        n3928 = case shown="True" w9002 {
          tunnel: w9003 -> [w9016 w9053]
          tunnel: [w9012 w9035] -> w8982
          tunnel: w8997 -> [w9018 w9045]
          tunnel: w8996 -> [w9021 w9046]
          tunnel: [w9011 w9034] -> w8995
          tunnel: w8994 -> [_ w9066]
          tunnel: w8993 -> [_ w9065]
          tunnel: w8992 -> [_ w9062]
          tunnel: w8991 -> [_ w9061]
          tunnel: w8990 -> [_ w9058]
          tunnel: w8983 -> [_ _]
          tunnel: [w9016 w9042] -> w8981
          tunnel: w8980 -> [_ w9041]
          tunnel: w8979 -> [_ w9040]
          tunnel: w8978 -> [_ w9039]
          tunnel: w8977 -> [_ w9038]
          frame False {
            n3929 = call-dynamic "Read Acq_prevstate.vi"("error in (no error)"=w9018, "Acquisition in"=w9021) -> ("error out"=w9017:errorcluster, "Acq_prevstate"=w9019:u32, "Acquisition out"=w9020:refnum<class "Acquisition.lvclass">)  [unwired: 7 in]
            n3930 = call-dynamic "Write Acq_state.vi"("error in (no error)"=w9017, "Acq_state"=w9019, "Acquisition in"=w9020) -> ("error out"=w9006:errorcluster, "Acquisition out"=w9010:refnum<class "Acquisition.lvclass">)  [unwired: 7 in]
            n3931 = call-dynamic "Read enabled.vi"("error in (no error)"=w9006, "Server in"=w9010) -> ("error out"=w9005:errorcluster, "enabled"=w9004:bool, "Server out"=w9009:refnum<class "Acquisition.lvclass">)  [unwired: 7 in]
            n3932 = call-dynamic "Read Channel.vi"("error in (no error)"=w9005, "Acquisition in"=w9009) -> ("error out"=w9007:errorcluster, "Channel.lvclass"=w9008:refnum<class "Channel.lvclass">, "Acquisition out"=w9014:refnum<class "Acquisition.lvclass">)  [unwired: 7 in]
            n3933 = case shown="True" w9004 {
              tunnel: w9008 -> [w9023 w9033]
              tunnel: [w9023 w9031] -> w9013
              tunnel: w9007 -> [w9022 w9028]
              tunnel: [w9022 w9026] -> w9015
              frame False {
              }
              frame True {
                n3934 = call-dynamic "Read State Machine.vi"("error in (no error)"=w9028, "Device in"=w9033) -> ("error out"=w9024:errorcluster, "State Machine.lvclass"=w9025:refnum<class "State Machine.lvclass">, "Device out"=w9032:refnum<class "Channel.lvclass">)  [unwired: 7 in]
                n3935 = call "Next State.vi"("error in (no error)"=w9024, "New_State"=96, "State Machine in"=w9025) -> ("error out"=w9027:errorcluster, "State Machine out"=w9030:refnum<class "State Machine.lvclass">)  [unwired: 7 in]
                n3936 = call-dynamic "Write State Machine.vi"("error in (no error)"=w9027, "State Machine.lvclass"=w9030, "Device in"=w9032) -> ("error out"=w9026:errorcluster, "Device out"=w9031:refnum<class "Channel.lvclass">)  [unwired: 7 in]
              }
            }
            n3937 = call-dynamic "Write Channel.vi"("error in (no error)"=w9015, "Channel.lvclass"=w9013, "Acquisition in"=w9014) -> ("error out"=w9012:errorcluster, "Acquisition out"=w9011:refnum<class "Acquisition.lvclass">)  [unwired: 7 in]
          }
          frame True {
            # "obs type"
            # "suffix"
            # "object"
            n3938 = call "Read Instrument.lvclass.vi"("S4ACS_GUI in"=w9053) -> ("error out"=w9055:errorcluster, "Instrument.lvclass"=w9057:refnum<class "Instrument.lvclass">, "S4ACS_GUI out"=w9043:refnum<class "S4GUI.lvclass">)  [unwired: 8 in]
            n3939 = call "Read WPROT.vi"("error in (no error)"=w9055, "Instrument in"=w9057) -> ("error out"=w9054:errorcluster, "Opt_Selector.lvclass"=w9056:refnum<class "Opt_Selector.lvclass">)  [unwired: 7 in, 1 out]
            n3940 = call-dynamic "Read sequencia.vi"("error in (no error)"=w9054, "Opt_Selector in"=w9056) -> ()  [unwired: 7 in, 3 out]
            n3941 = case shown="\"FOCUS\"" w9041 {
              tunnel: [u32 271 ("Obs_state") u32 251 ("Obs_state")] -> w9047
              tunnel: w9045 -> [w9094 w9105]
              tunnel: [w9093 w9105] -> w9044
              tunnel: w9040 -> [w9101 _]
              tunnel: w9039 -> [w9100 _]
              tunnel: w9038 -> [w9099 _]
              tunnel: w9043 -> [w9092 w9104]
              tunnel: [w9091 w9104] -> w9042
              frame "FOCUS" {
                n3942 = call-dynamic "Read TelFocus.lvclass.vi"("error in (no error)"=w9094, "S4GUI in"=w9092) -> ("error out"=w9096:errorcluster, "TelFocus.lvclass"=w9098:refnum<class "TelFocus.lvclass">, "S4GUI out"=w9102:refnum<class "S4GUI.lvclass">)  [unwired: 7 in]
                n3943 = call-dynamic "LoadParam.vi"("#steps"=w9099, "error in (no error)"=w9096, "step"=w9100, "init"=w9101, "TelFocus in"=w9098) -> ("error out"=w9095:errorcluster, "TelFocus out"=w9097:refnum<class "TelFocus.lvclass">)  [unwired: 5 in]
                n3944 = call-dynamic "Write TelFocus.lvclass.vi"("error in (no error)"=w9095, "TelFocus.lvclass"=w9097, "S4GUI in"=w9102) -> ("error out"=w9093:errorcluster, "S4GUI out"=w9091:refnum<class "S4GUI.lvclass">)  [unwired: 7 in]
              }
              frame Default {
              }
            }
            n3945 = call-dynamic "Write Acq_state.vi"("error in (no error)"=w9044, "Acq_state"=w9047, "Acquisition in"=w9046) -> ("error out"=w9067:errorcluster, "Acquisition out"=w9068:refnum<class "Acquisition.lvclass">)  [unwired: 7 in]
            n3946 = call-dynamic "Read Channel.vi"("error in (no error)"=w9067, "Acquisition in"=w9068) -> ("error out"=w9069:errorcluster, "Channel.lvclass"=w9070:refnum<class "Channel.lvclass">, "Acquisition out"=w9077:refnum<class "Acquisition.lvclass">)  [unwired: 7 in]
            n3947 = call-dynamic "Read Interface.vi"("error in (no error)"=w9069, "Channel in"=w9070) -> ("error out"=w9089:errorcluster, "Interface.lvclass"=w9090:refnum<class "Interface.lvclass">, "Channel out"=w9088:refnum<class "Channel.lvclass">)  [unwired: 7 in]
            n3948 = property on="Start ch4" class="Bool"(error in=w9045, "DisabledEnum"=T12."Disabled and Grayed Out" ("Disabled")) -> ()  [unwired: 1 in, 2 out]
            n3949 = call "Write Exposure Time.vi"("error in (no error)"=w9089, "Exposure Time"="Exptime ch4", "Interface in"=w9090) -> ("error out"=w9049:errorcluster, "Interface out"=w9052:refnum<class "Interface.lvclass">)  [unwired: 7 in]
            n3950 = case shown="\"ZERO\"" w9041 {
              tunnel: w9052 -> [w9108 w9113]
              tunnel: [w9108 w9112] -> w9051
              tunnel: [w9107 w9111] -> w9050
              tunnel: w9049 -> [w9107 w9110]
              tunnel: "Exptime ch4" -> [_ w9109]
              frame "ZERO" {
              }
              frame Default {
                n3951 = call-dynamic "Write prev ExpTime.vi"("error in (no error)"=w9110, "prev ExpTime"=w9109, "Interface in"=w9113) -> ("error out"=w9111:errorcluster, "Interface out"=w9112:refnum<class "Interface.lvclass">)  [unwired: 7 in]
              }
            }
            n3952 = call-dynamic "Write # Index.vi"("error in (no error)"=w9050, "# Index"="Index ch4", "Interface in"=w9051) -> ("error out"=w9086:errorcluster, "Interface out"=w9087:refnum<class "Interface.lvclass">)  [unwired: 7 in]
            n3953 = call-dynamic "Write Suffix.vi"("error in (no error)"=w9086, "Suffix"=w9066, "Interface in"=w9087) -> ("error out"=w9085:errorcluster, "Interface out"=w9084:refnum<class "Interface.lvclass">)  [unwired: 7 in]
            n3954 = call-dynamic "Write ObsType.vi"("error in (no error)"=w9085, "ObsType"=w9062, "Interface in"=w9084) -> ("error out"=w9082:errorcluster, "Interface out"=w9083:refnum<class "Interface.lvclass">)  [unwired: 7 in]
            n3955 = call-dynamic "Write Object.vi"("error in (no error)"=w9082, "Object"=w9061, "Interface in"=w9083) -> ("error out"=w9081:errorcluster, "Interface out"=w9080:refnum<class "Interface.lvclass">)  [unwired: 7 in]
            n3956 = call-dynamic "Write Comments.vi"("error in (no error)"=w9081, "Comments"=w9065, "Interface in"=w9080) -> ("error out"=w9078:errorcluster, "Interface out"=w9079:refnum<class "Interface.lvclass">)  [unwired: 7 in]
            n3957 = call-dynamic "Write DS9.vi"("error in (no error)"=w9078, "DS9"="F", "Interface in"=w9079) -> ("error out"=w9059:errorcluster, "Interface out"=w9060:refnum<class "Interface.lvclass">)  [unwired: 7 in]
            n3958 = call-dynamic "Write Observer.vi"("error in (no error)"=w9059, "Observer"=w9058, "Interface in"=w9060) -> ("error out"=w9063:errorcluster, "Interface out"=w9064:refnum<class "Interface.lvclass">)  [unwired: 7 in]
            n3959 = property on="Exposure Time ch4" class="Slide (strict)"("Scale.Maximum"="Exptime ch4", "Scale.Minimum"=0.0 ("Scale.Range:Minimum")) -> ()  [unwired: 2 in, 2 out]
            n3960 = call-dynamic "Write Interface.vi"("error in (no error)"=w9063, "Interface.lvclass"=w9064, "Channel in"=w9088) -> ("error out"=w9071:errorcluster, "Channel out"=w9072:refnum<class "Channel.lvclass">)  [unwired: 7 in]
            n3961 = call-dynamic "Write Channel.vi"("error in (no error)"=w9071, "Channel.lvclass"=w9072, "Acquisition in"=w9077) -> ("error out"=w9036:errorcluster, "Acquisition out"=w9037:refnum<class "Acquisition.lvclass">)  [unwired: 7 in]
            n3962 = call-dynamic "CalcCubeDuration.vi"("error in (no error)"=w9036, "Acquisition in"=w9037) -> ("error out"=w9035:errorcluster, "Acquisition out"=w9034:refnum<class "Acquisition.lvclass">)  [unwired: 8 in]
          }
        }
        n3963 = call-dynamic "Write AcquisitionD.vi"("error in (no error)"=w8982, "Acquisition.lvclass"=w8995, "S4ACS_GUI in"=w8981) -> ("error out"=w8973:errorcluster, "S4ACS_GUI out"=w8975:refnum<class "S4GUI.lvclass">)  [unwired: 7 in]
        n3964 = call-dynamic "Write User Event.vi"("error in (no error)"=w8973, "User Event"="START ASYNC CH4", "S4GUI in"=w8975) -> ("error out"=w8972:errorcluster, "S4GUI out"=w8974:refnum<class "S4GUI.lvclass">)  [unwired: 7 in]
      }
      event "Exptime ch1": Value Change {
        n3965 = event-data() -> ("NewVal"=w9118:dbl)  [unwired: 1 in]
        n3966 = call-dynamic "Read AcquisitionA.vi"("error in (no error)"=w9117, "S4ACS_GUI in"=w9116) -> ("error out"=w9132:errorcluster, "Acquisition.lvclass"=w9133:refnum<class "Acquisition.lvclass">, "S4ACS_GUI out"=w9130:refnum<class "S4GUI.lvclass">)  [unwired: 7 in]
        n3967 = call-dynamic "Read Channel.vi"("error in (no error)"=w9132, "Acquisition in"=w9133) -> ("error out"=w9121:errorcluster, "Channel.lvclass"=w9122:refnum<class "Channel.lvclass">, "Acquisition out"=w9123:refnum<class "Acquisition.lvclass">)  [unwired: 7 in]
        n3968 = call-dynamic "Read Interface.vi"("error in (no error)"=w9121, "Channel in"=w9122) -> ("error out"=w9127:errorcluster, "Interface.lvclass"=w9128:refnum<class "Interface.lvclass">, "Channel out"=w9126:refnum<class "Channel.lvclass">)  [unwired: 7 in]
        n3969 = call "Write Exposure Time.vi"("error in (no error)"=w9127, "Exposure Time"=w9118, "Interface in"=w9128) -> ("error out"=w9119:errorcluster, "Interface out"=w9120:refnum<class "Interface.lvclass">)  [unwired: 7 in]
        n3970 = call-dynamic "Write Interface.vi"("error in (no error)"=w9119, "Interface.lvclass"=w9120, "Channel in"=w9126) -> ("error out"=w9125:errorcluster, "Channel out"=w9124:refnum<class "Channel.lvclass">)  [unwired: 7 in]
        n3971 = call-dynamic "Write Channel.vi"("error in (no error)"=w9125, "Channel.lvclass"=w9124, "Acquisition in"=w9123) -> ("error out"=w9129:errorcluster, "Acquisition out"=w9131:refnum<class "Acquisition.lvclass">)  [unwired: 7 in]
        n3972 = call-dynamic "Write AcquisitionA.vi"("error in (no error)"=w9129, "Acquisition.lvclass"=w9131, "S4ACS_GUI in"=w9130) -> ("error out"=w9115:errorcluster, "S4ACS_GUI out"=w9114:refnum<class "S4GUI.lvclass">)  [unwired: 7 in]
      }
      event "Exptime ch2": Value Change {
        n3973 = event-data() -> ("NewVal"=w9138:dbl)  [unwired: 1 in]
        n3974 = call "Read AcquisitionB.vi"("error in (no error)"=w9137, "S4ACS_GUI in"=w9136) -> ("error out"=w9152:errorcluster, "Acquisition.lvclass"=w9153:refnum<class "Acquisition.lvclass">, "S4ACS_GUI out"=w9150:refnum<class "S4GUI.lvclass">)  [unwired: 7 in]
        n3975 = call-dynamic "Read Channel.vi"("error in (no error)"=w9152, "Acquisition in"=w9153) -> ("error out"=w9141:errorcluster, "Channel.lvclass"=w9142:refnum<class "Channel.lvclass">, "Acquisition out"=w9143:refnum<class "Acquisition.lvclass">)  [unwired: 7 in]
        n3976 = call-dynamic "Read Interface.vi"("error in (no error)"=w9141, "Channel in"=w9142) -> ("error out"=w9147:errorcluster, "Interface.lvclass"=w9148:refnum<class "Interface.lvclass">, "Channel out"=w9146:refnum<class "Channel.lvclass">)  [unwired: 7 in]
        n3977 = call "Write Exposure Time.vi"("error in (no error)"=w9147, "Exposure Time"=w9138, "Interface in"=w9148) -> ("error out"=w9139:errorcluster, "Interface out"=w9140:refnum<class "Interface.lvclass">)  [unwired: 7 in]
        n3978 = call-dynamic "Write Interface.vi"("error in (no error)"=w9139, "Interface.lvclass"=w9140, "Channel in"=w9146) -> ("error out"=w9145:errorcluster, "Channel out"=w9144:refnum<class "Channel.lvclass">)  [unwired: 7 in]
        n3979 = call-dynamic "Write Channel.vi"("error in (no error)"=w9145, "Channel.lvclass"=w9144, "Acquisition in"=w9143) -> ("error out"=w9149:errorcluster, "Acquisition out"=w9151:refnum<class "Acquisition.lvclass">)  [unwired: 7 in]
        n3980 = call "Write AcquisitionB.vi"("error in (no error)"=w9149, "Acquisition.lvclass"=w9151, "S4ACS_GUI in"=w9150) -> ("error out"=w9135:errorcluster, "S4ACS_GUI out"=w9134:refnum<class "S4GUI.lvclass">)  [unwired: 7 in]
      }
      event "Exptime ch3": Value Change {
        n3981 = event-data() -> ("NewVal"=w9158:dbl)  [unwired: 1 in]
        n3982 = call-dynamic "Read AcquisitionC.vi"("error in (no error)"=w9157, "S4ACS_GUI in"=w9156) -> ("error out"=w9172:errorcluster, "Acquisition.lvclass"=w9173:refnum<class "Acquisition.lvclass">, "S4ACS_GUI out"=w9170:refnum<class "S4GUI.lvclass">)  [unwired: 7 in]
        n3983 = call-dynamic "Read Channel.vi"("error in (no error)"=w9172, "Acquisition in"=w9173) -> ("error out"=w9161:errorcluster, "Channel.lvclass"=w9162:refnum<class "Channel.lvclass">, "Acquisition out"=w9163:refnum<class "Acquisition.lvclass">)  [unwired: 7 in]
        n3984 = call-dynamic "Read Interface.vi"("error in (no error)"=w9161, "Channel in"=w9162) -> ("error out"=w9167:errorcluster, "Interface.lvclass"=w9168:refnum<class "Interface.lvclass">, "Channel out"=w9166:refnum<class "Channel.lvclass">)  [unwired: 7 in]
        n3985 = call "Write Exposure Time.vi"("error in (no error)"=w9167, "Exposure Time"=w9158, "Interface in"=w9168) -> ("error out"=w9159:errorcluster, "Interface out"=w9160:refnum<class "Interface.lvclass">)  [unwired: 7 in]
        n3986 = call-dynamic "Write Interface.vi"("error in (no error)"=w9159, "Interface.lvclass"=w9160, "Channel in"=w9166) -> ("error out"=w9165:errorcluster, "Channel out"=w9164:refnum<class "Channel.lvclass">)  [unwired: 7 in]
        n3987 = call-dynamic "Write Channel.vi"("error in (no error)"=w9165, "Channel.lvclass"=w9164, "Acquisition in"=w9163) -> ("error out"=w9169:errorcluster, "Acquisition out"=w9171:refnum<class "Acquisition.lvclass">)  [unwired: 7 in]
